vi "Drive Encoder (RAW to Final).vi"(1 "encoderRAW[]":dbl[](array[numeric])) -> (0 "finalEncoder[]":dbl[](array[numeric]))   [LabVIEW 2018]
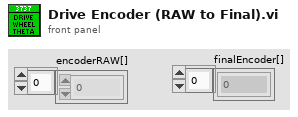
[diagram p1: front panel]
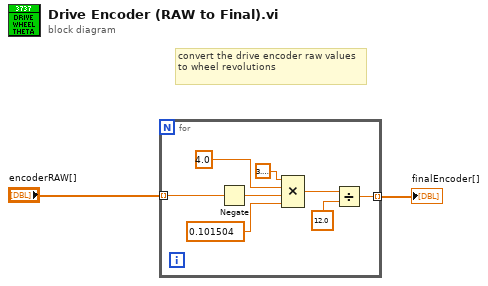
[diagram p0: block diagram]
diagram:
  # "convert the drive encoder raw values to wheel revolutions"
  n1 = for {
    tunnel: "encoderRAW[]" -> [w10] mode=indexing
    tunnel: [w3] -> w1 mode=indexing
    n2 = Negate(x=w10) -> (-x=w8:dbl)
    n3 = Compound Arithmetic op=MULTIPLY(3.141592653589793, 4.0 ("x"), w8, 0.101504 ("y")) -> (w5:dbl)
    n4 = Divide(x=w5, y=12.0) -> (x/y=w3:dbl)
  }
  "finalEncoder[]" <- w1
